vi "Format Channel to String.vi"(8 "error in":errorcluster, 11 "6700 in":refnum<class "6700.lvclass">) -> (0 "error out":errorcluster, 3 "6700 out":refnum<class "6700.lvclass">)   [LabVIEW 2018, in "6700.lvlib" / "6700.lvclass"]
uses:
  6700.lvclass
  6700.lvclass/6700.ctl
  builds/Power_Supply.lvlibp/Power Supply.lvclass
  C:/Users/Ron.Dexter.LUMINARTECH/Desktop/builds/Power_Supply.lvlibp/Power Supply.lvclass
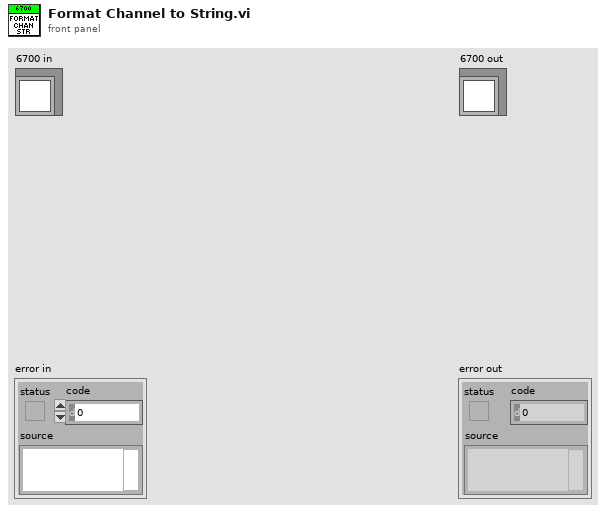
[diagram p1: front panel]
types:
  T1 = typedef "Power_Supply.lvlibp/Channel List.ctl" = enum16{"Channel 1", "Channel 2", "Channel 3", "Channel 4"}
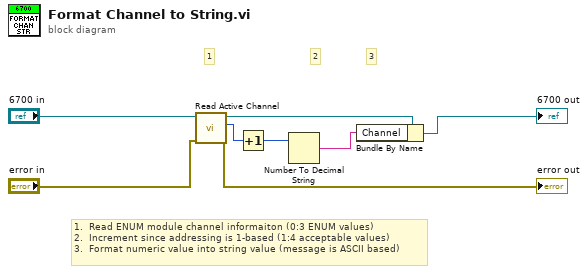
[diagram p0: block diagram]
diagram:
  # "1.  Read ENUM module channel informaiton (0:3 ENUM values)\n2.  Increment since addressing is 1-based (1:4 acceptable values)\n3.  Format numeric value into string value (message is ASCII based)"
  # "3"
  # "2"
  # "1"
  n1 = call "Read Active Channel.vi"("error in (no error)"="error in", "Power Supply in"="6700 in") -> ("error out"=→"error out":errorcluster, "Active Channel"=w5:T1, "Power Supply out"=w7:refnum<class "6700.lvclass">)  [unwired: 7 in]
  n2 = Increment(x=w5) -> (x+1=w6:T1)
  n3 = Number To Decimal String(number=w6) -> (decimal integer string=w1:string)  [unwired: 1 in]
  n4 = Bundle By Name(cluster=w7, "Channel"=w1) -> (→"6700 out":refnum<class "6700.lvclass">)
